vi "time.double_to_seconds-nanos.vi"(10 "Time (s)":dbl) -> (2 "Seconds Nanos":cluster{"seconds":i32, "nanos":i32})   [LabVIEW 2020, in "Nominal Client.lvclass"]
uses:
  Nominal Client.lvclass
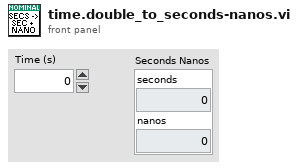
[diagram p1: front panel]
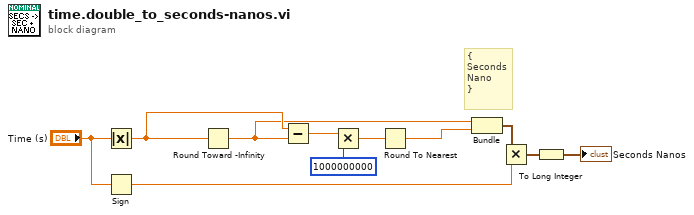
[diagram p0: block diagram]
diagram:
  # "{\nSeconds\nNano\n}"
  n1 = Absolute Value(x="Time (s)") -> (abs(x)=w6:dbl)
  n2 = Sign(1:"Time (s)") -> (0:w7:dbl)
  n3 = Round Toward -Infinity(1:w6) -> (0:w5:dbl)
  n4 = Subtract(x=w6, y=w5) -> (x-y=w11:dbl)
  n5 = Multiply(x=w11, y=1000000000) -> (x*y=w10:dbl)
  n6 = Round To Nearest(number=w10) -> (nearest integer value=w4:dbl)
  n7 = Bundle(w5, w4) -> (w3:cluster{dbl, dbl})  [unwired: 1 in]
  n8 = Multiply(x=w3, y=w7) -> (x*y=w2:cluster{dbl, dbl})
  n9 = To Long Integer(number=w2) -> (32bit integer=→"Seconds Nanos":cluster{i32, i32})
